vi "SERIAL_DecodeAHRSUpdatePacket.vi"(8 "error in":errorcluster, 10 "Buffer":string) -> (0 "error out":errorcluster, 3 "AHSR Data Packet":T4)   [LabVIEW 2014, in "navX-MXP IMU.lvlib"]
uses:
  navX-MXP IMU.lvlib
  COMMON/TypeDefs/Data TypeDefs/navX YPRH Data.ctl
  COMMON/TypeDefs/Data TypeDefs/navX Vector Data.ctl
  COMMON/TypeDefs/Data TypeDefs/navX Quaternion Data.ctl
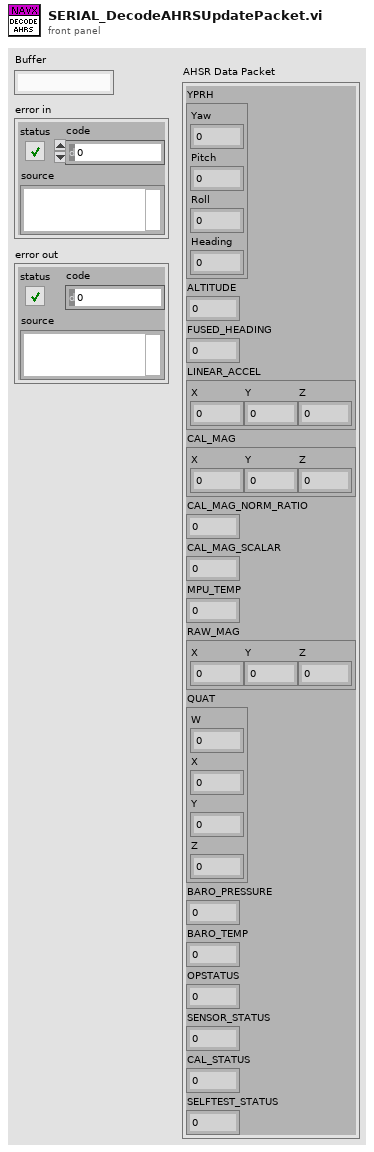
[diagram p1: front panel]
types:
  T1 = typedef "navX-MXP IMU.lvlib/navX YPRH Data.ctl" = cluster{"Yaw":dbl, "Pitch":dbl, "Roll":dbl, "Heading":dbl}
  T2 = typedef "navX-MXP IMU.lvlib/navX Vector Data.ctl" = cluster{"X":dbl, "Y":dbl, "Z":dbl}
  T3 = typedef "navX-MXP IMU.lvlib/navX Quaternion Data.ctl" = cluster{"W":dbl, "X":dbl, "Y":dbl, "Z":dbl}
  T4 = cluster{"YPRH":T1, "ALTITUDE":dbl, "FUSED_HEADING":dbl, "LINEAR_ACCEL":T2, "CAL_MAG":T2, "CAL_MAG_NORM_RATIO":dbl, "CAL_MAG_SCALAR":i32, "MPU_TEMP":dbl, "RAW_MAG":T2, "QUAT":T3, "BARO_PRESSURE":dbl, "BARO_TEMP":dbl, "OPSTATUS":i32, "SENSOR_STATUS":i32, "CAL_STATUS":i32, "SELFTEST_STATUS":i32}
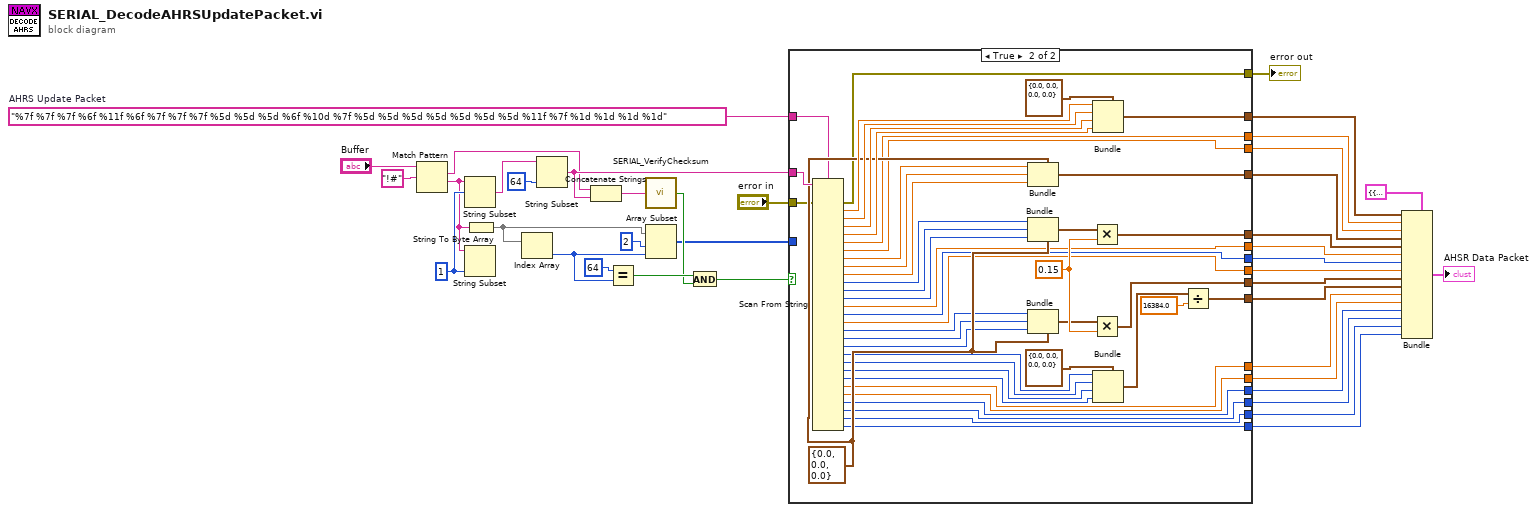
[diagram p0: block diagram]
diagram:
  w8 = 1 ("length (rest)")
  w27 = "%7f %7f %7f %6f %11f %6f %7f %7f %7f %5d %5d %5d %6f %10d %7f %5d %5d %5d %5d %5d %5d %5d %11f %7f %1d %1d %1d %1d"  # AHRS Update Packet
  n1 = Match Pattern(string="Buffer", regular expression="!#") -> (match substring=w7:string, after substring=w6:string)  [unwired: 1 in, 2 out]
  n2 = String Subset(string=w6, offset (0)=w8) -> (substring=w2:string)  [unwired: 1 in]
  n3 = String Subset(string=w6, length (rest)=w8) -> ()  [unwired: 1 in, 1 out]
  n4 = String To Byte Array(string=w6) -> (unsigned byte array=w5:u8[])
  n5 = Index Array(array=w5) -> (element=w1:u8)  [unwired: 1 in]
  n6 = String Subset(string=w2, length (rest)=64 ("length (rest)")) -> (substring=w30:string)  [unwired: 1 in]
  n7 = Concatenate Strings(w7, w30) -> (w32:string)
  n8 = Equal?(x=64, y=w1) -> (x = y?=w35:bool)
  n9 = call "SERIAL_VerifyChecksum.vi"("Content"=w32) -> ("Valid Checksum"=w33:bool)
  n10 = Array Subset(array=w5, index=2, length=w1) -> (w3:u8[])
  n11 = And(x=w35, y=w33) -> (x .and. y?=w31:bool)
  n12 = case shown="True" w31 {
    tunnel: w30 -> [_ w84]
    tunnel: [_ w58] -> w24
    tunnel: [_ w57] -> w21
    tunnel: [_ w56] -> w20
    tunnel: [_ w55] -> w16
    tunnel: [_ w54] -> w15
    tunnel: [_ w53] -> w23
    tunnel: [_ w52] -> w22
    tunnel: [_ w51] -> w19
    tunnel: [_ w50] -> w18
    tunnel: [_ w49] -> w17
    tunnel: [_ w48] -> w14
    tunnel: [_ w47] -> w13
    tunnel: [_ w46] -> w11
    tunnel: [_ w45] -> w12
    tunnel: [_ w44] -> w10
    tunnel: [_ w43] -> w9
    tunnel: [w39 w42] -> w29
    tunnel: "error in" -> [w39 w41]
    tunnel: w27 -> [_ w40]
    tunnel: w3 -> [_ _]
    frame False {
    }
    frame True {
      w67 = 0.15 ("y")
      w78 = T2 {"X"=0.0, "Y"=0.0, "Z"=0.0} ("Vector")
      n13 = Scan From String(format string=w40, input string=w84, error in=w41) -> (error out=w42:errorcluster, output 1=w83:dbl, output 2=w82:dbl, output 3=w81:dbl, output 4=w80:dbl, output 5=w53:dbl, output 6=w52:dbl, output 7=w77:dbl, output 8=w76:dbl, output 9=w75:dbl, output 10=w74:i32, output 11=w73:i32, output 12=w72:i32, output 13=w51:dbl, output 14=w50:i32, output 15=w49:dbl, output 16=w70:i32, output 17=w69:i32, output 18=w68:i32, output 19=w64:i32, output 20=w63:i32, output 21=w62:i32, output 22=w61:i32, output 23=w48:dbl, output 24=w47:dbl, output 25=w46:i32, output 26=w45:i32, output 27=w44:i32, output 28=w43:i32)  [unwired: 29 in, 2 out]
      n14 = Bundle(cluster=w78, "X"=w77, "Y"=w76, "Z"=w75) -> (w57:T2)
      n15 = Bundle(cluster=w78, "X"=w74, "Y"=w73, "Z"=w72) -> (w71:T2)
      n16 = Bundle(cluster=w78, "X"=w70, "Y"=w69, "Z"=w68) -> (w66:T2)
      n17 = Multiply(x=w71, y=w67) -> (x*y=w56:T2)
      n18 = Multiply(x=w66, y=w67) -> (x*y=w55:T2)
      n19 = Bundle(cluster=T1 {"Yaw"=0.0, "Pitch"=0.0, "Roll"=0.0, "Heading"=0.0} ("YPRH"), "Yaw"=w83, "Pitch"=w82, "Roll"=w81, "Heading"=w80) -> (w58:T1)
      n20 = Bundle(cluster=T3 {"W"=0.0, "X"=0.0, "Y"=0.0, "Z"=0.0} ("Quaternion"), "W"=w64, "X"=w63, "Y"=w62, "Z"=w61) -> (w59:T3)
      n21 = Divide(x=w59, y=16384.0) -> (x/y=w54:T3)
    }
  }
  "error out" <- w29
  n22 = Bundle(cluster=T4 {"YPRH"={"Yaw"=0.0, "Pitch"=0.0, "Roll"=0.0, "Heading"=0.0}, "ALTITUDE"=0.0, "FUSED_HEADING"=0.0, "LINEAR_ACCEL"={"X"=0.0, "Y"=0.0, "Z"=0.0}, "CAL_MAG"={"X"=0.0, "Y"=0.0, "Z"=0.0}, "CAL_MAG_NORM_RATIO"=0.0, "CAL_MAG_SCALAR"=0, "MPU_TEMP"=0.0, "RAW_MAG"={"X"=0.0, "Y"=0.0, "Z"=0.0}, "QUAT"={"W"=0.0, "X"=0.0, "Y"=0.0, "Z"=0.0}, "BARO_PRESSURE"=0.0, "BARO_TEMP"=0.0, "OPSTATUS"=0, "SENSOR_STATUS"=0, "CAL_STATUS"=0, "SELFTEST_STATUS"=0} ("AHSR Data Packet"), "YPRH"=w24, "ALTITUDE"=w23, "FUSED_HEADING"=w22, "LINEAR_ACCEL"=w21, "CAL_MAG"=w20, "CAL_MAG_NORM_RATIO"=w19, "CAL_MAG_SCALAR"=w18, "MPU_TEMP"=w17, "RAW_MAG"=w16, "QUAT"=w15, "BARO_PRESSURE"=w14, "BARO_TEMP"=w13, "OPSTATUS"=w11, "SENSOR_STATUS"=w12, "CAL_STATUS"=w10, "SELFTEST_STATUS"=w9) -> (→"AHSR Data Packet":T4)
